vi "CSM - Convert Error to Argument.vi"(4 "error in (no error)":errorcluster) -> (1 "Arguments":string)   [LabVIEW 2020, in "Communicable State Machine.lvlib"]
uses:
  Communicable State Machine.lvlib
  CSM - Keywords.vi
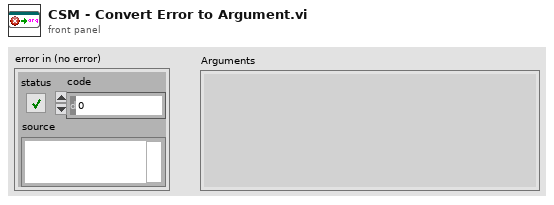
[diagram p1: front panel]
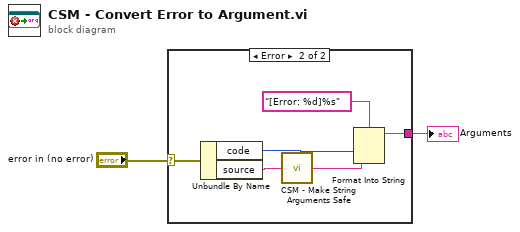
[diagram p0: block diagram]
diagram:
  n1 = case shown="Error" "error in (no error)" {
    selector: "error in (no error)" -> [_ w7]
    tunnel: [_ w8] -> w2
    frame No Error {
    }
    frame Error {
      n2 = Unbundle By Name(w7) -> ("code"=w4:i32, "source"=w3:string)
      n3 = call "CSM - Make String Arguments Safe.vi"("Argurment String"=w3) -> ("Safe Argurment String"=w5:string)  [unwired: 8 in]
      n4 = Format Into String(format string="[Error: %d]%s", w4, w5) -> (resulting string=w8:string)  [unwired: 2 in, 1 out]
    }
  }
  "Arguments" <- w2
